vi "Get client handle.vi"(8 "error in (no error)":errorcluster, 9 "headers":T1[](array[typedef]), 11 "REST Client in":refnum<class "REST Client_JKI.lvclass">) -> (0 "error out":errorcluster, 1 "headers out":T1[](array[typedef]), 2 "Client Handle":T2, 3 "REST Client out":refnum<class "REST Client_JKI.lvclass">)   [LabVIEW 2018, in "REST Client.lvlib" / "REST Client_JKI.lvclass"]
uses:
  REST Client_JKI.lvclass
  <vilib>/httpClient/ClientHandle.ctl
  REST Client/HTTP Header.ctl
  REST Client_JKI.lvclass/REST Client_JKI.ctl
  <vilib>/httpClient/LabVIEWHTTPClient.lvlib
  REST Client/REST Client.lvclass
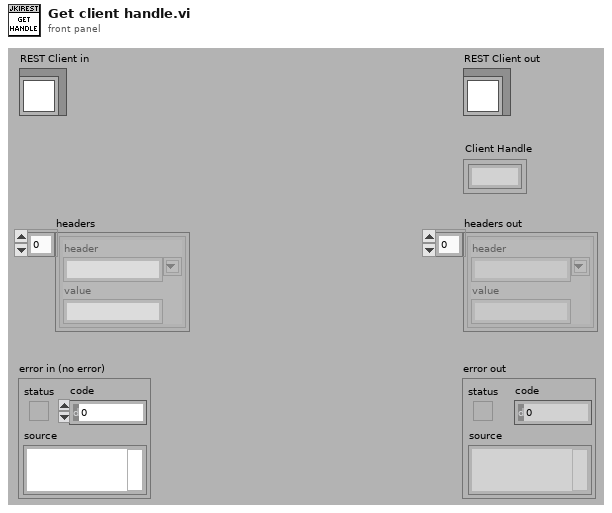
[diagram p1: front panel]
types:
  T1 = typedef "REST Client.lvlib/REST Client.lvclass/HTTP Header.ctl" = cluster{"header":string, "value":string}
  T2 = typedef "LabVIEWHTTPClient.lvlib/ClientHandle.ctl" = refnum<k1>
  T3 = cluster{"client handle out":T2, "Default Headers ([JSON])":T1[]}
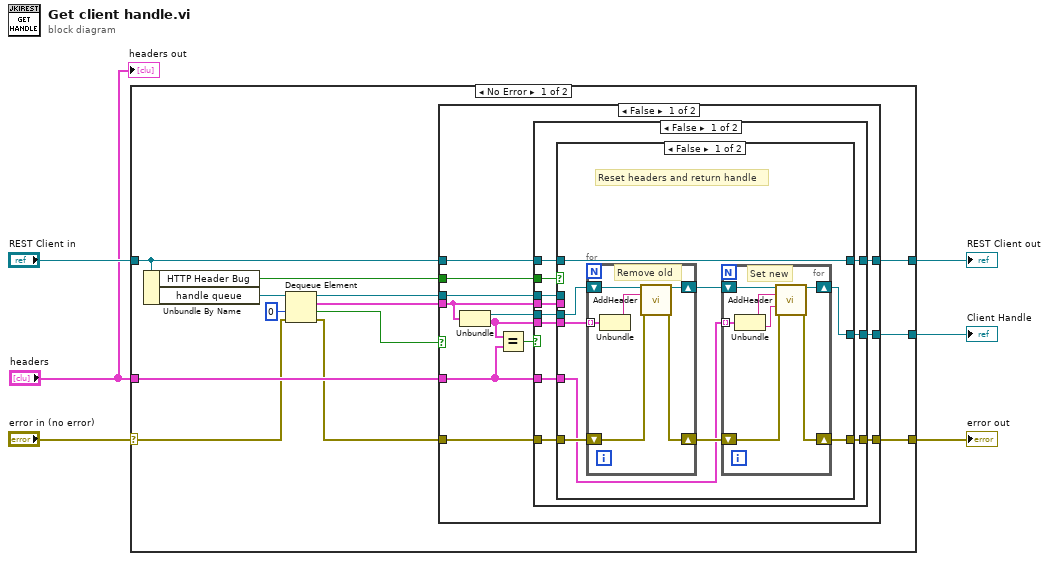
[diagram p0: block diagram]
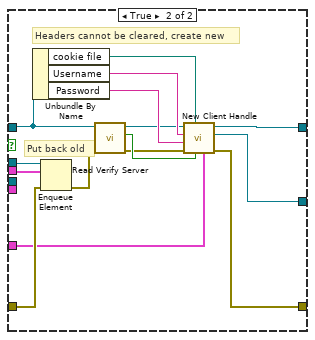
[diagram p2: hidden frame]
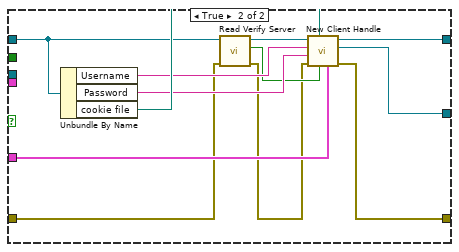
[diagram p4: hidden frame]
diagram:
  n1 = case shown="No Error" "error in (no error)" {
    selector: "error in (no error)" -> [w12 w95]
    tunnel: [w16 w95] -> w5
    tunnel: [w19 w96] -> w3
    tunnel: "REST Client in" -> [w15 w96]
    tunnel: [w17 _] -> w2
    tunnel: "headers" -> [w18 _]
    frame No Error {
      n2 = Unbundle By Name(w15) -> ("HTTP Header Bug"=w8:bool, "handle queue"=w14:refnum<queue>)
      n3 = Dequeue Element(queue=w14, timeout in ms (-1)=0, error in (no error)=w12) -> (queue out=w7:refnum<queue>, element=w9:T3, timed out?=w10:bool, error out=w11:errorcluster)
      n4 = case shown="False" w10 {
        tunnel: [w22 w94] -> w19
        tunnel: w18 -> [w28 w90]
        tunnel: [w27 w89] -> w17
        tunnel: [w26 w88] -> w16
        tunnel: w15 -> [w23 w87]
        tunnel: w11 -> [w25 w84]
        tunnel: w9 -> [w20 _]
        tunnel: w8 -> [w24 _]
        tunnel: w7 -> [w21 _]
        frame False {
          n5 = Unbundle(w20) -> ("client handle out"=w30:T2, "Default Headers ([JSON])"=w29:T1[])
          n6 = Equal?(x=w29, y=w28) -> (x = y?=w31:bool)
          n7 = case shown="False" w31 {
            tunnel: w30 -> [w33 w82]
            tunnel: w29 -> [w32 _]
            tunnel: w28 -> [w36 _]
            tunnel: [w34 w82] -> w27
            tunnel: [w35 w81] -> w26
            tunnel: w25 -> [w38 w81]
            tunnel: w24 -> [w42 _]
            tunnel: w23 -> [w41 w80]
            tunnel: [w37 w80] -> w22
            tunnel: w21 -> [w40 _]
            tunnel: w20 -> [w39 _]
            frame False {
              n8 = case shown="False" w42 {
                tunnel: w41 -> [w51 w75]
                tunnel: w40 -> [_ w79]
                tunnel: w39 -> [_ w78]
                tunnel: w38 -> [w48 w77]
                tunnel: [w51 w76] -> w37
                tunnel: w36 -> [w43 w71]
                tunnel: [w45 w70] -> w35
                tunnel: [w46 w69] -> w34
                tunnel: w33 -> [w50 _]
                tunnel: w32 -> [w49 _]
                frame False {
                  # "Reset headers and return handle"
                  n9 = for {
                    shift-right: [w62] -> w44
                    shift-left: w48 -> [w61]
                    shift-right: [w63] -> w47
                    shift-left: w50 -> [w64]
                    tunnel: w49 -> [w60] mode=indexing
                    # "Remove old"
                    n10 = Unbundle(w60) -> ("header"=w59:string)  [unwired: 1 out]
                    n11 = call <vilib>:"AddHeader.vi"("client handle"=w64, "header"=w59, "error in (no error)"=w61) -> ("client handle out"=w63:T2, "error out"=w62:errorcluster)  [unwired: 11 in]
                  }
                  n12 = for {
                    shift-right: [w56] -> w45
                    shift-left: w44 -> [w55]
                    shift-right: [w57] -> w46
                    shift-left: w47 -> [w58]
                    tunnel: w43 -> [w54] mode=indexing
                    # "Set new"
                    n13 = Unbundle(w54) -> ("header"=w53:string, "value"=w52:string)
                    n14 = call <vilib>:"AddHeader.vi"("client handle"=w58, "header"=w53, "value"=w52, "error in (no error)"=w55) -> ("client handle out"=w57:T2, "error out"=w56:errorcluster)  [unwired: 10 in]
                  }
                }
                frame True {
                  # "Put back old"
                  # "Headers cannot be cleared, create new"
                  n15 = Unbundle By Name(w75) -> ("cookie file"=w74:path, "Username"=w73:string, "Password"=w72:string)
                  n16 = Enqueue Element(queue=w79, element=w78, error in (no error)=w77) -> (error out=w66:errorcluster)  [unwired: 1 in, 2 out]
                  n17 = call-dynamic "Read Verify Server.vi"("error in (no error)"=w66, "REST Client in"=w75) -> ("error out"=w65:errorcluster, "Verify Server"=w67:bool, "REST Client out"=w68:refnum<class "REST Client_JKI.lvclass">)  [unwired: 7 in]
                  n18 = call "New Client Handle.vi"("headers"=w71, "verify server(true)"=w67, "cookie file"=w74, "error in (no error)"=w65, "password"=w72, "username"=w73, "REST Client in"=w68) -> ("error out"=w70:errorcluster, "client handle out"=w69:T2, "REST Client out"=w76:refnum<class "REST Client_JKI.lvclass">)  [unwired: 2 in]
                }
              }
            }
            frame True {
              # "Use existing handle"
            }
          }
        }
        frame True {
          n19 = Unbundle By Name(w87) -> ("Username"=w92:string, "Password"=w91:string, "cookie file"=w93:path)
          n20 = call-dynamic "Read Verify Server.vi"("error in (no error)"=w84, "REST Client in"=w87) -> ("error out"=w83:errorcluster, "Verify Server"=w85:bool, "REST Client out"=w86:refnum<class "REST Client_JKI.lvclass">)  [unwired: 7 in]
          n21 = call "New Client Handle.vi"("headers"=w90, "verify server(true)"=w85, "cookie file"=w93, "error in (no error)"=w83, "password"=w91, "username"=w92, "REST Client in"=w86) -> ("error out"=w88:errorcluster, "client handle out"=w89:T2, "REST Client out"=w94:refnum<class "REST Client_JKI.lvclass">)  [unwired: 2 in]
        }
      }
    }
    frame Error {
    }
  }
  "error out" <- w5
  "REST Client out" <- w3
  "Client Handle" <- w2
  "headers out" <- "headers"
